vi "SC TCP Unflatten SequenceRun.vi"(8 "error in":errorcluster, 11 "Response JSON":string) -> (0 "error out":errorcluster, 3 "Return":T1)   [LabVIEW 2018]
uses:
  SC TCP SequenceRun.ctl
  SC TCP StepResult.ctl
panel:
  out "Command Completed":bool
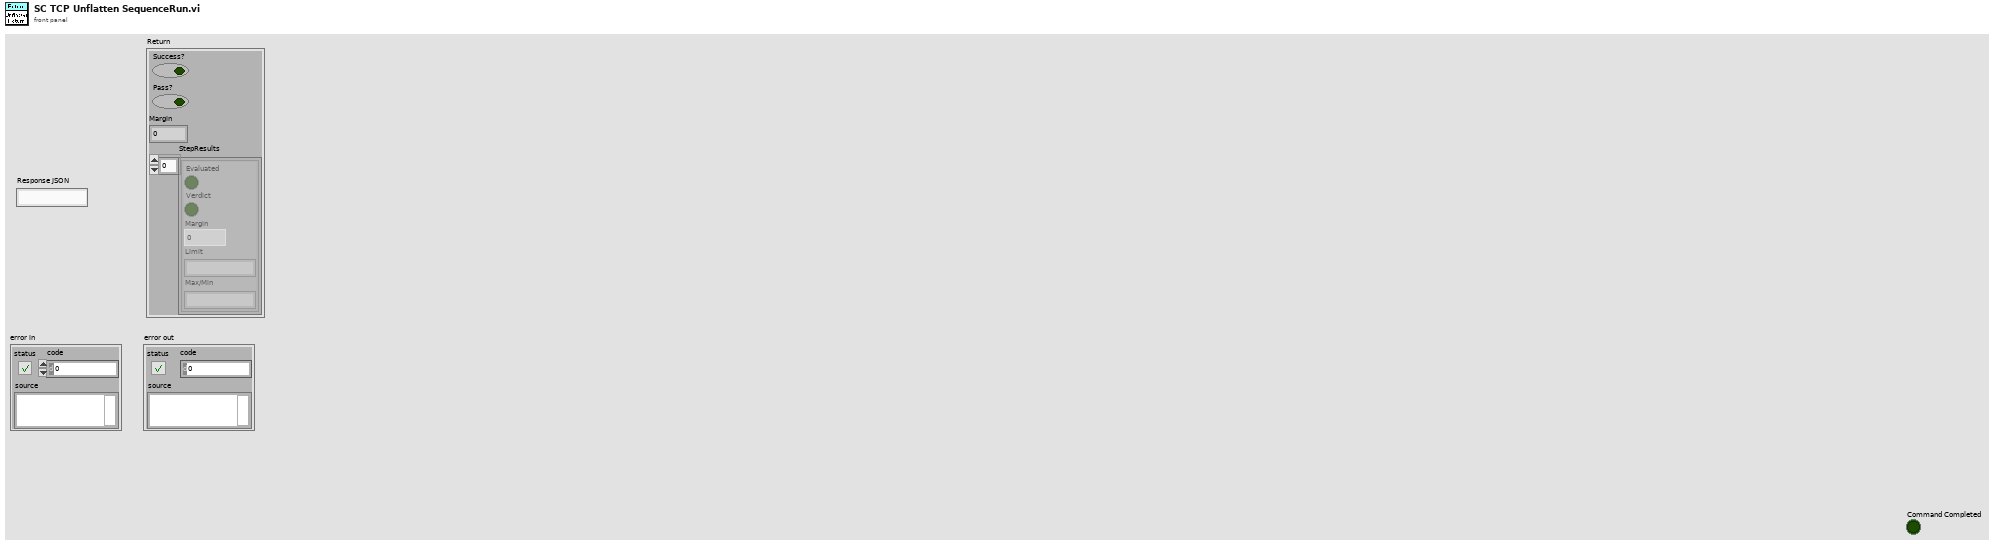
[diagram p1: front panel]
types:
  T1 = typedef "SC TCP SequenceRun.ctl" = cluster{"Success?":bool, "Pass?":bool, "Margin":dbl, "StepResults":T2[]}
  T2 = typedef "SC TCP StepResult.ctl" = cluster{"Evaluated":bool, "Verdict":bool, "Margin":dbl, "Limit":string, "Max/Min":string}
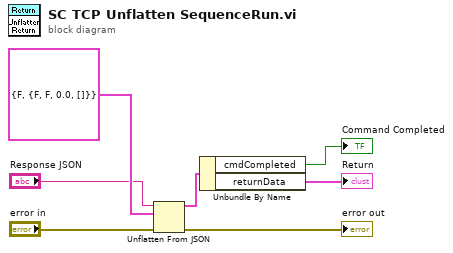
[diagram p0: block diagram]
diagram:
  n1 = Unflatten From JSON(JSON string="Response JSON", type and defaults=cluster{"cmdCompleted":bool, "returnData":T1} {"cmdCompleted"=FALSE, "returnData"={"Success?"=FALSE, "Pass?"=FALSE, "Margin"=0.0, "StepResults"=[]}} ("Response Details"), error in (no error)="error in") -> (value=w6:cluster{"cmdCompleted":bool, "returnData":T1}, error out=→"error out":errorcluster)  [unwired: 4 in]
  n2 = Unbundle By Name(w6) -> ("cmdCompleted"=→"Command Completed":bool, "returnData"=→"Return":T1)
